vi "Pressure_Monitor.vi"(11 "VISA resource name":refnum<visa-resource-name>) -> (0 "Error at segmenting output":errorcluster, 1 "Error at VISA Read":errorcluster, 3 "Flow readout":dbl)   [LabVIEW 2015]
uses:
  <vilib>/Utility/config.llb/Read Key (I32).vi
  <vilib>/Utility/config.llb/NI_LVConfig.lvlib
panel:
  out "Waveform Chart 2":dbl(graph)
  out "date/time string 2":string
  out "current time 2":timestamp
  out "decimal integer string":string
  out "remaining string":string
  out "read buffer":string
  out "result":bool
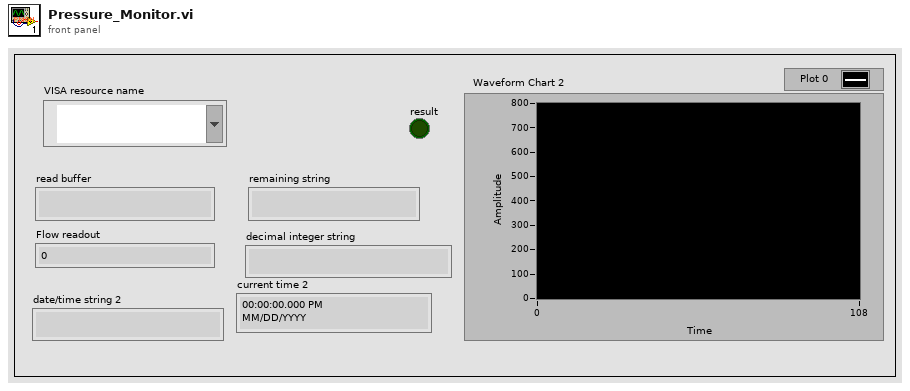
[diagram p1: front panel]
types:
  T1 = typedef "NI_LVConfig.lvlib/Config Data RefNum.ctl" = refnum<k1>
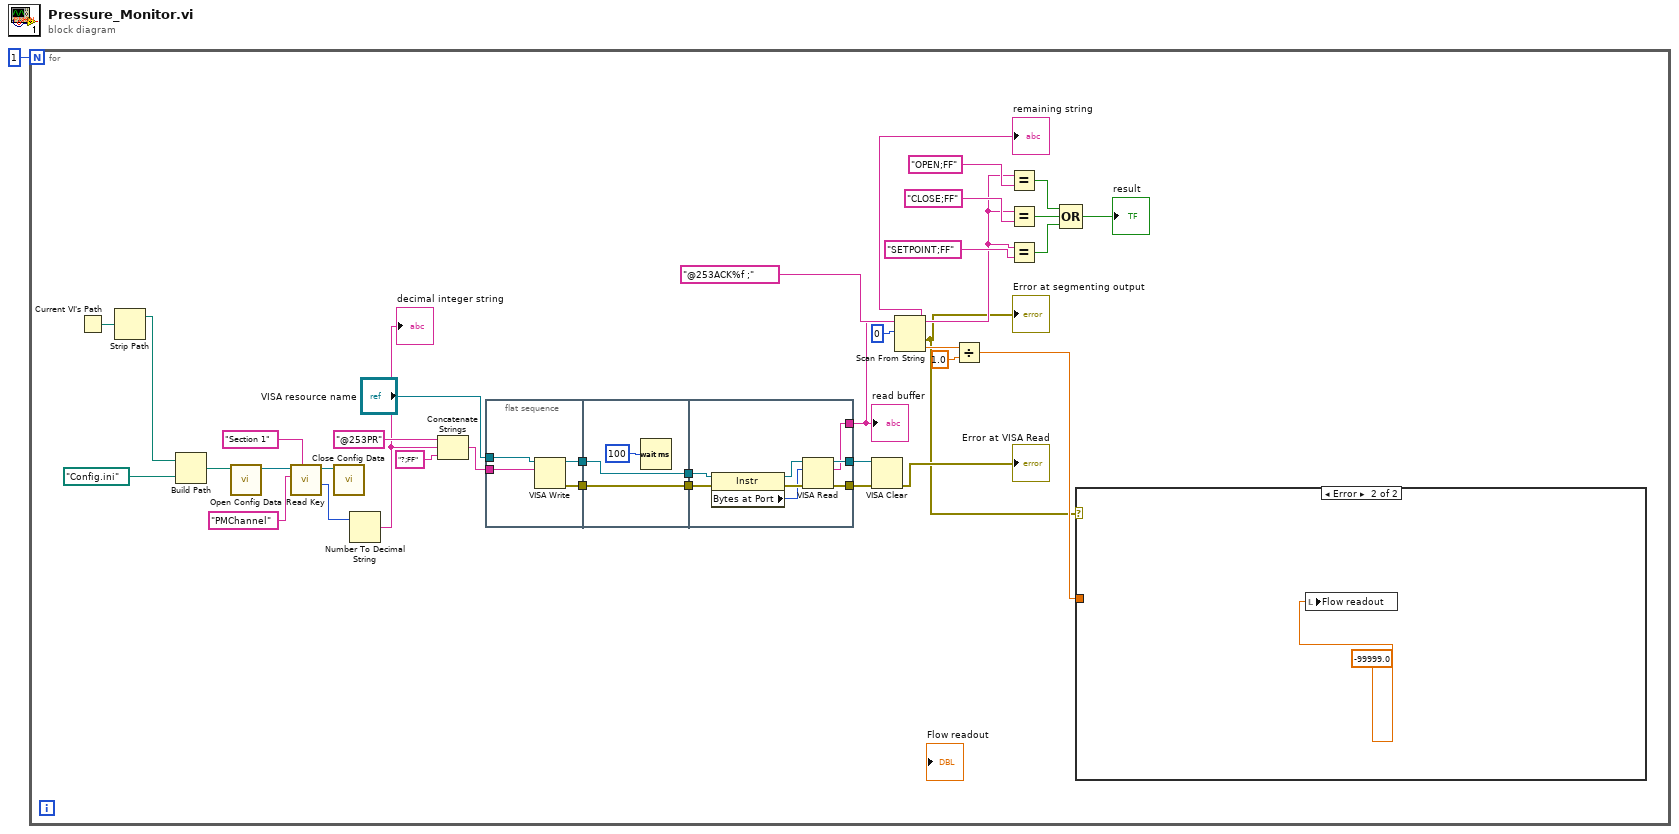
[diagram p0: block diagram]
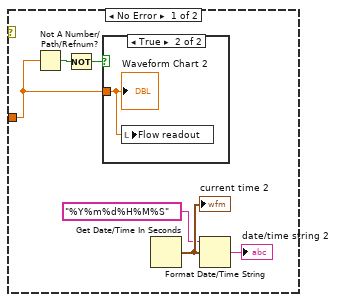
[diagram p2: hidden frame]
diagram:
  n1 = for {
    N: 1 -> [_]
    n2 = Current VI's Path() -> (path=w3:path)
    n3 = Strip Path(path=w3) -> (stripped path=w2:path)  [unwired: 1 out]
    n4 = Build Path(base path=w2, name or relative path=path "Config.ini" ("default name")) -> (appended path=w26:path)
    n5 = call <vilib>:"Open Config Data.vi"("configuration file path"=w26) -> ("refnum"=w33:T1)  [unwired: 8 in, 2 out]
    n6 = call-poly <vilib>:"Read Key.vi"("section"="Section 1", "key"="PMChannel", "refnum"=w33) -> ("value"=w30:i32, "refnum out"=w31:T1)  [unwired: 5 in, 2 out]
    n7 = call <vilib>:"Close Config Data.vi"("refnum"=w31) -> ()  [unwired: 9 in, 2 out]
    n8 = Number To Decimal String(number=w30) -> (decimal integer string=w28:string)  [unwired: 1 in]
    "decimal integer string" <- w28
    n9 = Concatenate Strings("@253PR" ("string"), w28, "?;FF" ("string")) -> (w12:string)
    n10 = flat-sequence {
      tunnel: w12 -> [w41]
      tunnel: "VISA resource name" -> [w40]
      tunnel: [w39] -> w10
      tunnel: [w38] -> w8
      tunnel: w10 -> [w43]
      tunnel: [w43] -> w9
      tunnel: w8 -> [w42]
      tunnel: [w42] -> w7
      tunnel: w9 -> [w49]
      tunnel: w7 -> [w48]
      tunnel: [w47] -> w6
      tunnel: [w46] -> w4
      tunnel: [w45] -> w5
      frame #0 {
        n11 = VISA Write(VISA resource name=w40, write buffer=w41) -> (VISA resource name out=w39:refnum<visa-resource-name>, error out=w38:errorcluster)  [unwired: 1 in, 1 out]
      }
      frame #1 {
        n12 = Wait (ms)(milliseconds to wait=u32 100) -> ()  [unwired: 1 out]
      }
      frame #2 {
        n13 = property class="Instr"(reference=w49, error in=w48) -> (reference out=w50:refnum<visa-resource-name>, error out=w52:errorcluster, "Bytes at Port"=w51:u32)
        n14 = VISA Read(VISA resource name=w50, byte count=w51, error in (no error)=w52) -> (VISA resource name out=w47:refnum<visa-resource-name>, read buffer=w45:string, error out=w46:errorcluster)  [unwired: 1 out]
      }
    }
    n15 = VISA Clear(VISA resource name=w6, error in (no error)=w4) -> (error out=→"Error at VISA Read":errorcluster)  [unwired: 1 out]
    n16 = Scan From String(format string="@253ACK%f ;", input string=w5, initial scan location=u32 0) -> (remaining string=w16:string, error out=w13:errorcluster, output 1=w24:dbl)  [unwired: 2 in, 1 out]
    "Error at segmenting output" <- w13
    "remaining string" <- w16
    n17 = Divide(x=w24, y=1.0) -> (x/y=w23:dbl)
    n18 = Equal?(x=w16, y="OPEN;FF") -> (x = y?=w21:bool)
    n19 = Equal?(x=w16, y="CLOSE;FF") -> (x = y?=w20:bool)
    n20 = Equal?(x=w16, y="SETPOINT;FF") -> (x = y?=w17:bool)
    n21 = Compound Arithmetic op=OR(w21, w20, w17) -> (→"result":bool)
    n22 = case shown="Error" w13 {
      tunnel: w23 -> [w54 _]
      frame No Error {
        n23 = Not A Number/Path/Refnum?(number/path/refnum=w54) -> (NaN/Path/Refnum?=w56:bool)
        n24 = Not(x=w56) -> (.not. x?=w55:bool)
        n25 = case shown="True" w55 {
          tunnel: w54 -> [_ w59]
          frame False {
          }
          frame True {
            n26 = local write "Flow readout"(w59) -> ()
            "Waveform Chart 2" <- w59
          }
        }
        n27 = Get Date/Time In Seconds() -> (seconds since 1Jan1904=w58:timestamp)
        "current time 2" <- w58
        n28 = Format Date/Time String(time format string (%c)="%Y%m%d%H%M%S", seconds (now)=w58) -> (date/time string=→"date/time string 2":string)  [unwired: 1 in]
      }
      frame Error {
        n29 = local write "Flow readout"(-99999.0) -> ()
      }
    }
    "read buffer" <- w5
  }
